vi "HWT_UNITHERM_Proc_LocalUpdate.vi"(8 "Error In":errorcluster, 10 "Data":string, 11 "Command":string) -> (0 "Error Out":errorcluster)   [LabVIEW 2015]
uses:
  S2C_UNITHERM_Proc_Globals.vi
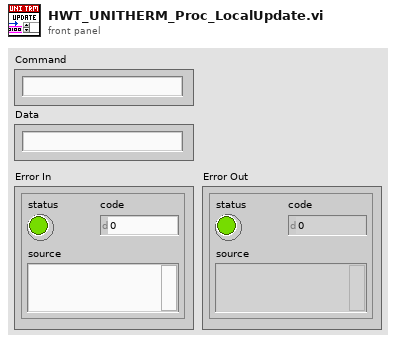
[diagram p1: front panel]
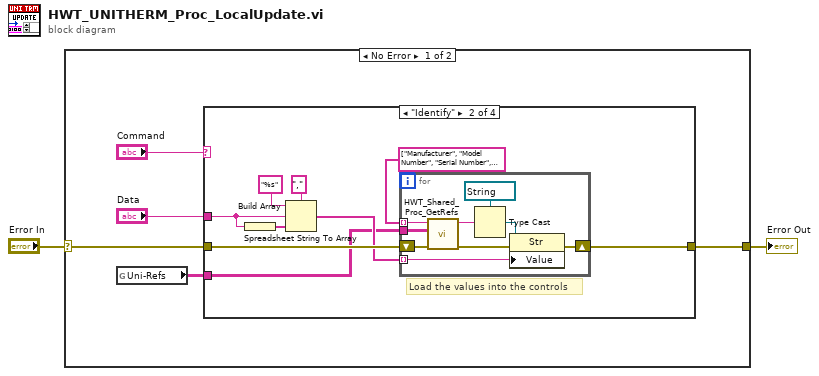
[diagram p0: block diagram]
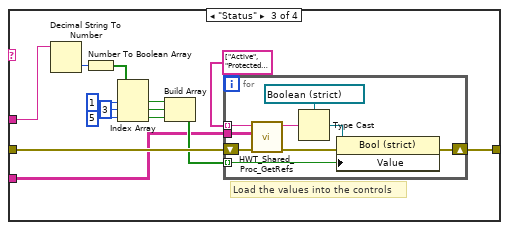
[diagram p3: hidden frame]
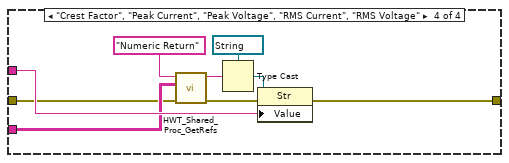
[diagram p4: hidden frame]
diagram:
  n1 = case shown="No Error" "Error In" {
    selector: "Error In" -> [w6 w59]
    tunnel: [w4 w59] -> w1
    frame No Error {
      n2 = global read "S2C_UNITHERM_Proc_Globals.vi" "Uni-Refs"() -> (w3:string[][])
      n3 = case shown="\"Identify\"" "Command" {
        tunnel: w6 -> [w8 w13 w40 w53]
        tunnel: "Data" -> [_ w14 w36 w55]
        tunnel: [w8 w10 w38 w56] -> w4
        tunnel: w3 -> [_ w9 w27 w54]
        frame "Other", Default {
        }
        frame "Identify" {
          # "Load the values into the controls"
          n4 = Build Array(w14) -> (w15:string[])
          n5 = Spreadsheet String To Array(delimiter (Tab)=",", format string="%s", spreadsheet string=w14, array type (2D Dbl)=w15) -> (array=w12:string[])
          n6 = for {
            tunnel: w12 -> [w24] mode=indexing
            tunnel: string[] ["Manufacturer", "Model Number", "Serial Number", "Firmware Version"] -> [w20] mode=indexing
            shift-right: [w23] -> w10
            shift-left: w13 -> [w18]
            tunnel: w9 -> [w19]
            n7 = call "HWT_Shared_Proc_GetRefs.vi"("Error In"=w18, "Refs"=w19, "Label"=w20) -> ("Error Out"=w22:errorcluster, "Reference"=w21:string)  [unwired: 7 in]
            n8 = Type Cast(type=refnum<vi> refnum ("Enum"), x=w21) -> (*(type *) &x=w25:refnum<vi>)
            n9 = property class="Str"(reference=w25, error in=w22, "Value"=w24) -> (error out=w23:errorcluster)  [unwired: 1 out]
          }
        }
        frame "Status" {
          # "Load the values into the controls"
          n10 = Decimal String To Number(string=w36) -> (number=w37:i32)  [unwired: 2 in, 1 out]
          n11 = Number To Boolean Array(number=w37) -> (Boolean array=w29:bool[])
          n12 = Index Array(array=w29, index #1=1 ("index"), index #2=3 ("index"), index #3=5 ("index")) -> (element #1=w30:bool, element #2=w31:bool, element #3=w32:bool)
          n13 = Build Array(w30, w31, w32) -> (w28:bool[])
          n14 = for {
            tunnel: w28 -> [w48] mode=indexing
            tunnel: string[] ["Active", "Protected", "Disconnected"] -> [w45] mode=indexing
            shift-right: [w47] -> w38
            shift-left: w40 -> [w43]
            tunnel: w27 -> [w44]
            n15 = call "HWT_Shared_Proc_GetRefs.vi"("Error In"=w43, "Refs"=w44, "Label"=w45) -> ("Error Out"=w41:errorcluster, "Reference"=w42:string)  [unwired: 7 in]
            n16 = Type Cast(type=refnum<vi> refnum ("Boolean"), x=w42) -> (*(type *) &x=w49:refnum<vi>)
            n17 = property class="Bool (strict)"(reference=w49, error in=w41, "Value"=w48) -> (error out=w47:errorcluster)  [unwired: 1 out]
          }
        }
        frame "Crest Factor", "Peak Current", "Peak Voltage", "RMS Current", "RMS Voltage" {
          n18 = call "HWT_Shared_Proc_GetRefs.vi"("Error In"=w53, "Refs"=w54, "Label"="Numeric Return") -> ("Error Out"=w52:errorcluster, "Reference"=w51:string)  [unwired: 7 in]
          n19 = Type Cast(type=refnum<vi> refnum ("Enum"), x=w51) -> (*(type *) &x=w57:refnum<vi>)
          n20 = property class="Str"(reference=w57, error in=w52, "Value"=w55) -> (error out=w56:errorcluster)  [unwired: 1 out]
        }
      }
    }
    frame Error {
    }
  }
  "Error Out" <- w1
